vi "Execute.vi"(8 "error in":errorcluster, 11 "Set QO2 in":refnum<class "Set QO2.lvclass">) -> (0 "error out":errorcluster, 1 "Next Step?":bool, 2 "MSG":string, 3 "Set QO2 out":refnum<class "Set QO2.lvclass">)   [LabVIEW 2015, in "Set QO2.lvclass"]
uses:
  Set QO2.lvclass
  Controls/MFC Address.ctl
  Reusable/Sequence/STEPS/LEAVES/Double/Switch DBL.lvclass/Switch DBL.ctl
  Reusable/Sequence/STEPS/LEAVES/Double/Read val.vi
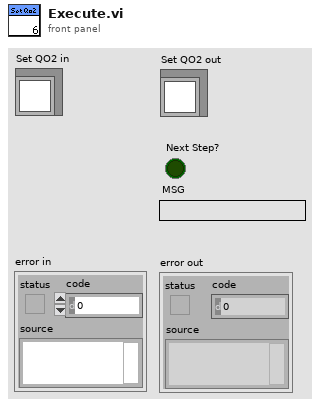
[diagram p1: front panel]
types:
  T1 = typedef "MFC Address.ctl" = enum16{"CRDS Purge", "CRDS Thermodenuded", "CRDS Dry", "CRDS Med RH", "CRDS High RH", "PAS Ch 1", "PAS Ch 2", "PAS Ch3", "PAS Ch 4", "PAS Ch 5", "CLAP", "O3", "Pinlet"}
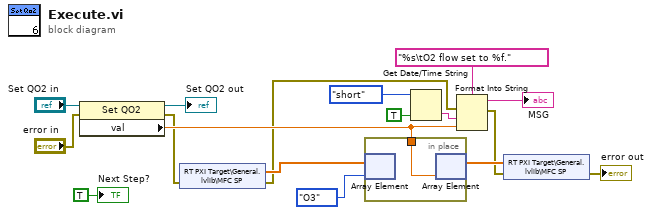
[diagram p0: block diagram]
diagram:
  n1 = property class="Set QO2"(reference="Set QO2 in", error in="error in") -> (reference out=→"Set QO2 out":refnum<class "Set QO2.lvclass">, error out=w6:errorcluster, "val"=w10:dbl)
  n2 = shared-variable "RT PXI Target\\General.lvlib\\MFC SP"(error in=w6) -> (w11:sgl[], error out=w5:errorcluster)
  n3 = in-place {
    in-place-border: w10 -> [w18]
    n4 = in-place-array #1(w11, MFC_Address."O3" ("Controllers")) -> ()  [unwired: 1 out]
    n5 = in-place-array #1(w18) -> (w9:sgl[])  [unwired: 1 out]
  }
  n6 = Get Date/Time String(date format (0)=enum16{"short", "long", "abbreviated"}."short", want seconds? (F)=TRUE) -> (time string=w13:string)  [unwired: 1 in, 1 out]
  n7 = Format Into String(format string="%s\tO2 flow set to %f.", error in=w5, w13, w10) -> (resulting string=→"MSG":string, error out=w4:errorcluster)  [unwired: 1 in]
  n8 = shared-variable "RT PXI Target\\General.lvlib\\MFC SP"(w9, error in=w4) -> (error out=→"error out":errorcluster)
  "Next Step?" <- TRUE ("Next Step?")
